vi "Pixy1Or2ObjectSelection.vi"(8 "Second Object":string, 9 "Empty?":bool, 11 "First Object":string) -> (0 "Y Axis Out":dbl, 2 "Width Out":dbl, 3 "X Axis Out":dbl)   [LabVIEW 2016]
panel:
  out "2 Y":dbl
  out "2 X":dbl
  out "1 Y":dbl
  out "1 X":dbl
  out "2 Height":dbl
  out "2 Width":dbl
  out "1 Height":dbl
  out "1 Width":dbl
  # "Select case depending\non whether or not two\nobjects are detected"
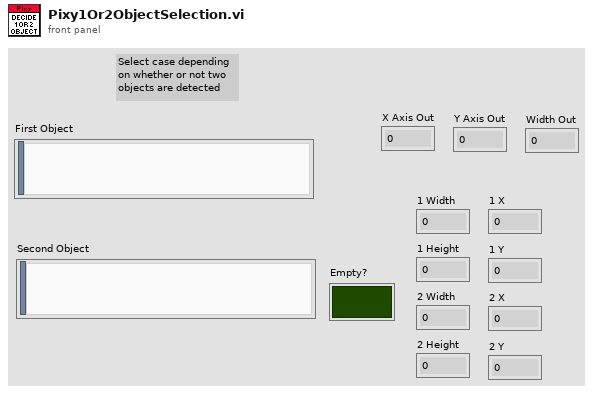
[diagram p1: front panel]
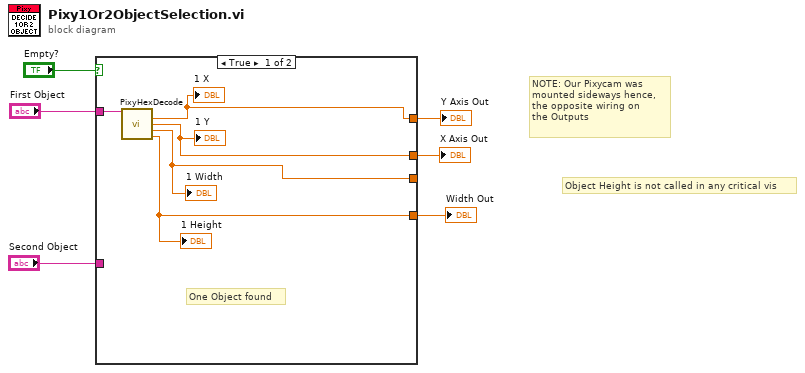
[diagram p0: block diagram]
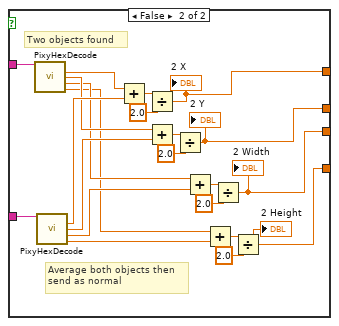
[diagram p2: hidden frame]
diagram:
  # "NOTE: Our Pixycam was\nmounted sideways hence,\nthe opposite wiring on\nthe Outputs"
  # "Object Height is not called in any critical vis"
  n1 = case shown="True" "Empty?" {
    tunnel: "First Object" -> [w11 w33]
    tunnel: [w9 w14] -> w4
    tunnel: [w10 w15] -> w1
    tunnel: "Second Object" -> [_ w32]
    tunnel: [w8 w13] -> _
    tunnel: [w7 w12] -> w2
    frame True {
      # "One Object found"
      n2 = call "PixyHexDecode.vi"("Object"=w11) -> ("X"=w7:dbl, "Y"=w9:dbl, "Width"=w8:dbl, "Height"=w10:dbl)  [unwired: 10 in, 1 out]
      "1 Width" <- w8
      "1 Height" <- w10
      "1 X" <- w7
      "1 Y" <- w9
    }
    frame False {
      # "Two objects found"
      # "Average both objects then\nsend as normal"
      n3 = call "PixyHexDecode.vi"("Object"=w33) -> ("X"=w23:dbl, "Y"=w21:dbl, "Width"=w19:dbl, "Height"=w17:dbl)  [unwired: 10 in, 1 out]
      n4 = call "PixyHexDecode.vi"("Object"=w32) -> ("X"=w22:dbl, "Y"=w20:dbl, "Width"=w18:dbl, "Height"=w16:dbl)  [unwired: 10 in, 1 out]
      n5 = Add(x=w23, y=w22) -> (x+y=w31:dbl)
      n6 = Divide(x=w31, y=2.0) -> (x/y=w12:dbl)
      "2 X" <- w12
      n7 = Add(x=w21, y=w20) -> (x+y=w29:dbl)
      n8 = Divide(x=w29, y=2.0) -> (x/y=w14:dbl)
      "2 Y" <- w14
      n9 = Add(x=w19, y=w18) -> (x+y=w27:dbl)
      n10 = Add(x=w17, y=w16) -> (x+y=w25:dbl)
      n11 = Divide(x=w27, y=2.0) -> (x/y=w13:dbl)
      "2 Width" <- w13
      n12 = Divide(x=w25, y=2.0) -> (x/y=w15:dbl)
      "2 Height" <- w15
    }
  }
  "X Axis Out" <- w4
  "Y Axis Out" <- w2
  "Width Out" <- w1
